vi "Format Z Position Data.vi"   [LabVIEW 2013]
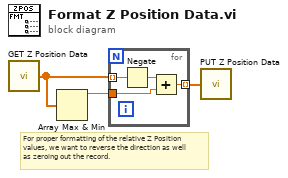
[diagram p0: block diagram]
diagram:
  # "For proper formatting of the relative Z Position\nvalues, we want to reverse the direction as well\nas zeroing out the record."
  n1 = call "GET Z Position Data.vi"() -> ("Z Position Data"=w3:dbl[])
  n2 = Array Max & Min(array=w3) -> (max value=w2:dbl)  [unwired: 3 out]
  n3 = for {
    tunnel: w3 -> [w7] mode=indexing
    tunnel: w2 -> [w5]
    tunnel: [w4] -> w1 mode=indexing
    n4 = Negate(x=w7) -> (-x=w6:dbl)
    n5 = Add(x=w6, y=w5) -> (x+y=w4:dbl)
  }
  n6 = call "PUT Z Position Data.vi"("Z Position Data"=w1) -> ()
